vi "32xx_VISA_Config_Serial_Port.vi"(0 "VISA resource name":refnum<visa-resource-name>="COM5" caption="Nom VISA In", 1 "timeout (10sec)":u32=10000 caption="timeout (10s)", 2 "termination char\n(0xA = '\\n' = LF)":u8=13 caption="car. de terminaison\n(0xA = 'n' = LF)" format="%.0x", 3 "Enable Termination\nChar (T)":bool caption="Activer caractère de \nterminaison (V)", 5 "baud rate (9600)":u32=9600 caption="débit en bauds (9600)", 7 "data bits (8)":u16=8 caption="bits de données (8)" min=5 max=8 step=1, 9 "parity (0:none)":enum16{"None", "Odd", "Even", "Mark", "Space"}(ring) caption="parité (0 : none)", 11 "error in (no error)":errorcluster caption="entrée d'erreur", 12 "stop bits (10: 1 bit)":u16(ring)=10 caption="bits de stop (10 : 1 bit)" items=["1.0"=10, "1.5"=15, "2.0"=20], 13 "flow control (0:none)":u16(ring) caption="contrôle de flux (0 : aucun)" items=["Aucun", "XON/XOFF", "RTS/CTS", "XON/XOFF & RTS/CTS", "DTR/DSR", "XON/XOFF & DTR/DSR"]) -> (4 "référence en sortie":refnum<visa-resource-name>="COM5" caption="Nom VISA Out", 15 "error out":errorcluster caption="sortie d'erreur")   [LabVIEW 2020]
doc: "Configuration du port série (Baud rate, data bits , etc..)"
panel:
  # "0xD= C.R"
  # "© 2020 elc CORPORATION.  \nALL RIGHTS RESERVED.."
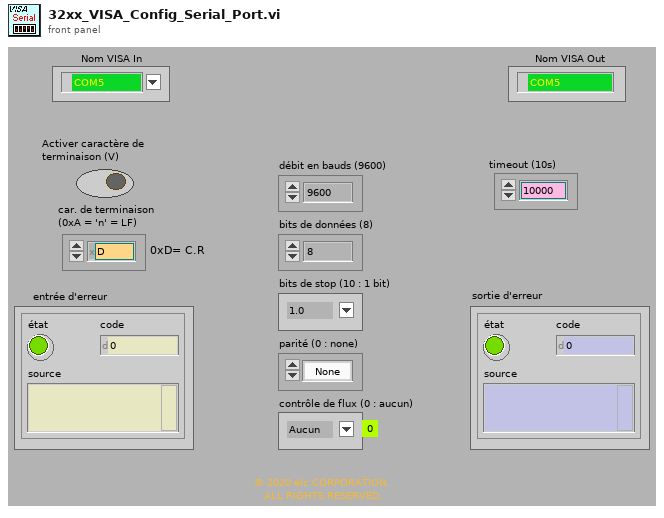
[diagram p1: front panel]
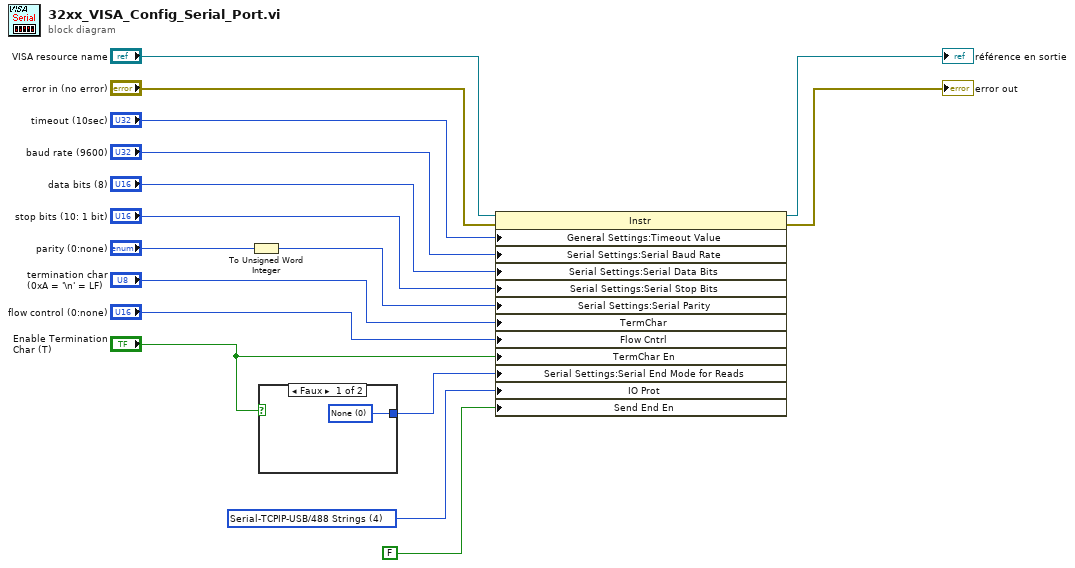
[diagram p0: block diagram]
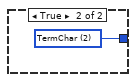
[diagram p2: hidden frame]
diagram:
  w2 = u16 4 items=["Normal"=1, "VXI/FDC"=2, "GPIB/HS488"=3, "Serial-TCPIP-USB/488 Strings"=4, "USBTMC/Vendor-Specific"=5] ("Message Based Settings:IO Protocol")
  n1 = To Unsigned Word Integer(number="parity (0:none)") -> (unsigned 16bit integer=w6:u16)
  n2 = case shown="Faux" "Enable Termination\nChar (T)" {
    tunnel: [w17 w18] -> w9
    frame False {
      w17 = u16 0 items=["None", "LastBit", "TermChar"] ("Serial Settings:Serial End Mode for Reads")
    }
    frame True {
      w18 = u16 2 items=["None", "LastBit", "TermChar"] ("Serial Settings:Serial End Mode for Reads")
    }
  }
  n3 = property class="Instr"(reference="VISA resource name", error in="error in (no error)", "General Settings:Timeout Value"="timeout (10sec)", "Serial Settings:Serial Baud Rate"="baud rate (9600)", "Serial Settings:Serial Data Bits"="data bits (8)", "Serial Settings:Serial Stop Bits"="stop bits (10: 1 bit)", "Serial Settings:Serial Parity"=w6, "TermChar"="termination char\n(0xA = '\\n' = LF)", "Flow Cntrl"="flow control (0:none)", "TermChar En"="Enable Termination\nChar (T)", "Serial Settings:Serial End Mode for Reads"=w9, "IO Prot"=w2, "Send End En"=FALSE ("Message Based Settings:Send End Enable")) -> (reference out=→"référence en sortie":refnum<visa-resource-name>, error out=→"error out":errorcluster)
